vi "image to RGB.vi"(3 "Numeric":i32, 5 "Y Resolution":i32, 7 "X Resolution":i32, 11 "image chiffrée":T1) -> (0 "blue out":u32[](array[numeric]), 1 "green out":u32[](array[numeric]), 2 "red out":u32[](array[numeric]))   [LabVIEW 2019]
uses:
  <vilib>/vision/Image Controls.llb/IMAQ Image.ctl
  <vilib>/vision/NI_Vision_Development_Module.lvlib
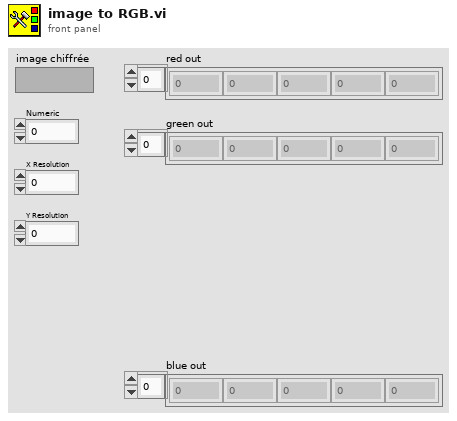
[diagram p1: front panel]
types:
  T1 = typedef "IMAQ Image.ctl" = refnum<image>
  T2 = cluster{"Red (or Hue) value":u8, "Green (or Sat) value":u8, "Blue (or Light or Val) value":u8}
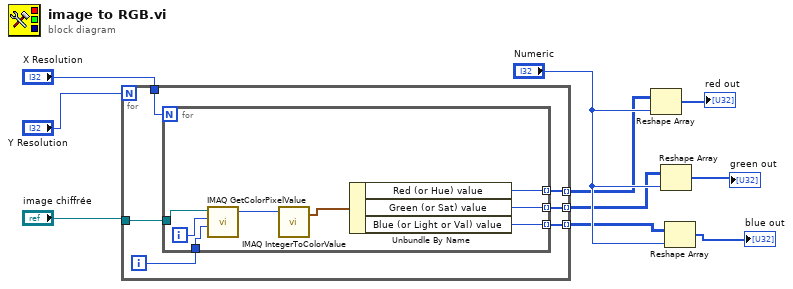
[diagram p0: block diagram]
diagram:
  n1 = for {
    N: "Y Resolution" -> [_]
    tunnel: "image chiffrée" -> [w16]
    tunnel: [w14] -> w1 mode=indexing
    tunnel: [w13] -> w3 mode=indexing
    tunnel: [w12] -> w2 mode=indexing
    tunnel: "X Resolution" -> [w11]
    i -> [w15]
    n2 = for {
      N: w11 -> [_]
      tunnel: w16 -> [w24]
      tunnel: w15 -> [w21]
      tunnel: [w20] -> w14 mode=indexing
      tunnel: [w19] -> w13 mode=indexing
      tunnel: [w18] -> w12 mode=indexing
      i -> [w17]
      n3 = call "IMAQ GetColorPixelValue"("Y Coordinate"=w21, "X Coordinate"=w17, "Image"=w24) -> ("Pixel Value (U32)"=w22:u32)  [unwired: 1 in, 2 out]
      n4 = call "IMAQ IntegerToColorValue"("U32 value"=w22) -> ("Color Value"=w23:T2)  [unwired: 4 in, 3 out]
      n5 = Unbundle By Name(w23) -> ("Red (or Hue) value"=w20:u8, "Green (or Sat) value"=w19:u8, "Blue (or Light or Val) value"=w18:u8)
    }
  }
  n6 = Reshape Array(w1, "Numeric") -> (→"red out":u8[])
  n7 = Reshape Array(w3, "Numeric") -> (→"green out":u8[])
  n8 = Reshape Array(w2, "Numeric") -> (→"blue out":u8[])
